vi "To Pretty String (Array).vi"(6 "pretty print? (T)":bool=TRUE, 7 "enable LabVIEW extensions? (T)":bool=TRUE, 8 "error in (no error)":errorcluster, 10 "indent":i32, 11 "JSON Value in":variant) -> (0 "error out":errorcluster, 3 "Pretty Print String":string)   [LabVIEW 2017, in "Advanced Variant Tools.lvlib"]
doc: "Pretty prints the given JSON data in an easier to read format."
uses:
  Advanced Variant Tools.lvlib
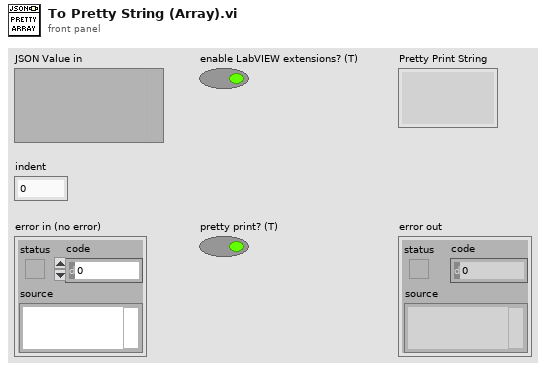
[diagram p1: front panel]
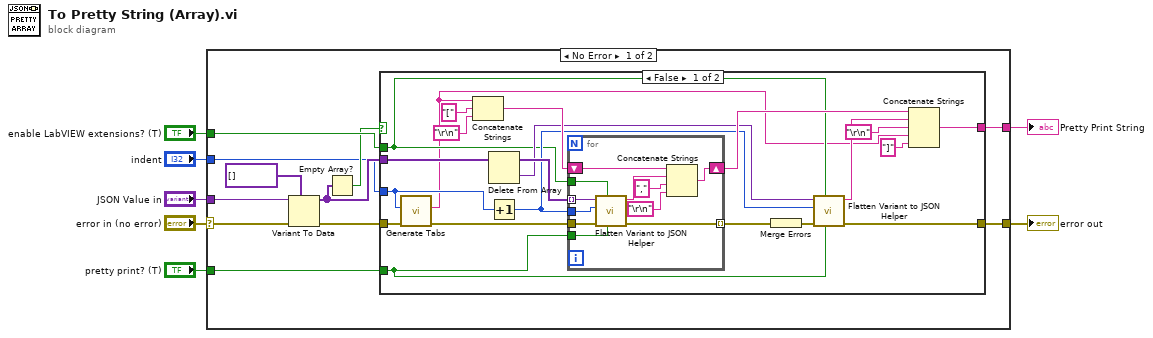
[diagram p0: block diagram]
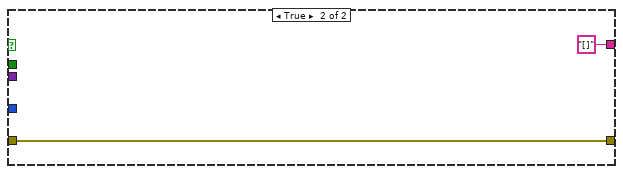
[diagram p2: hidden frame]
diagram:
  n1 = case shown="No Error" "error in (no error)" {
    selector: "error in (no error)" -> [w14 w53]
    tunnel: [w18 _] -> w7
    tunnel: [w17 w53] -> w6
    tunnel: "enable LabVIEW extensions? (T)" -> [w16 _]
    tunnel: "JSON Value in" -> [w15 _]
    tunnel: "indent" -> [w10 _]
    tunnel: "pretty print? (T)" -> [w9 _]
    frame No Error {
      n2 = Variant To Data(error in=w14, type=variant[] [], Variant=w15) -> (data=w11:variant[], error out=w13:errorcluster)
      n3 = Empty Array?(array=w11) -> (empty?=w12:bool)
      n4 = case shown="False" w12 {
        tunnel: [w39 "[]"] -> w18
        tunnel: [w24 w51] -> w17
        tunnel: w11 -> [w29 _]
        tunnel: w16 -> [w22 _]
        tunnel: w13 -> [w38 w51]
        tunnel: w10 -> [w37 _]
        tunnel: w9 -> [w23 _]
        frame False {
          n5 = call "Generate Tabs.vi"("error in (no error)"=w38, "indent"=w37) -> ("error out"=w35:errorcluster, "Tabs"=w19:string)  [unwired: 8 in]
          n6 = Concatenate Strings(w19, "[" ("string"), "\r\n") -> (w33:string)
          n7 = Delete From Array(array=w29) -> (deleted portion=w27:variant, array with subset deleted=w28:variant[])  [unwired: 2 in]
          n8 = Increment(x=w37) -> (x+1=w26:i32)
          n9 = for {
            tunnel: w28 -> [w50] mode=indexing
            tunnel: w26 -> [w49]
            tunnel: w35 -> [w48]
            shift-right: [w46] -> w32
            shift-left: w33 -> [w45]
            tunnel: [w44] -> w31 mode=indexing
            tunnel: w23 -> [w43]
            tunnel: w22 -> [w42]
            n10 = call "Flatten Variant to JSON Helper.vi"("pretty print? (T)"=w43, "enable LabVIEW extensions? (T)"=w42, "error in (no error)"=w48, "indent"=w49, "JSON Value in"=w50) -> ("error out"=w44:errorcluster, "String"=w47:string)  [unwired: 5 in]
            n11 = Concatenate Strings(w45, w47, "," ("string"), "\r\n") -> (w46:string)
          }
          n12 = Merge Errors(w31) -> (w25:errorcluster)
          n13 = call "Flatten Variant to JSON Helper.vi"("pretty print? (T)"=w23, "enable LabVIEW extensions? (T)"=w22, "error in (no error)"=w25, "indent"=w26, "JSON Value in"=w27) -> ("error out"=w24:errorcluster, "String"=w21:string)  [unwired: 5 in]
          n14 = Concatenate Strings(w32, w21, "\r\n", w19, "]" ("string")) -> (w39:string)
        }
        frame True {
        }
      }
    }
    frame Error {
    }
  }
  "error out" <- w6
  "Pretty Print String" <- w7
